vi "MGI VI Scripting Pattern.vi"   [LabVIEW 2016]
doc: "Pattern for scripting VI's to make them more organized and therefore readable.\n\nAuthor: David A. Moore\nsupport@mooregoodideas.com\nwww.mooregoodideas.com\n\nCopyright (c) 2013, Moore Good Ideas, Inc.\n\nAll rights reserved.\n\nRedistribution and use in source and binary forms, with or without modification, are permitted provided that the following conditions are met:\n\n * Redistributions of source code must retain the above copyright notice, this list of conditions and the following disclaimer.\n * Redistributions in binary form must reproduce the above copyright notice, this list of conditions and the following disclaimer in the documentation and/or other materials provided with the distribution.\n * Neither the name of Moore Good Ideas, Inc. nor the names of its contributors may be used to endorse or promote products derived from this software without specific prior written permission.\n\nTHIS SOFTWARE IS PROVIDED BY THE COPYRIGHT HOLDERS AND CONTRIBUTORS \"AS IS\" AND ANY EXPRESS OR IMPLIED WARRANTIES, INCLUDING, BUT NOT LIMITED TO, THE IMPLIED WARRANTIES OF MERCHANTABILITY AND FITNESS FOR A PARTICULAR PURPOSE ARE DISCLAIMED. IN NO EVENT SHALL THE COPYRIGHT OWNER OR CONTRIBUTORS BE LIABLE FOR ANY DIRECT, INDIRECT, INCIDENTAL, SPECIAL, EXEMPLARY, OR CONSEQUENTIAL DAMAGES (INCLUDING, BUT NOT LIMITED TO, PROCUREMENT OF SUBSTITUTE GOODS OR SERVICES; LOSS OF USE, DATA, OR PROFITS; OR BUSINESS INTERRUPTION) HOWEVER CAUSED AND ON ANY THEORY OF LIABILITY, WHETHER IN CONTRACT, STRICT LIABILITY, OR TORT (INCLUDING NEGLIGENCE OR OTHERWISE) ARISING IN ANY WAY OUT OF THE USE OF THIS SOFTWARE, EVEN IF ADVISED OF THE POSSIBILITY OF SUCH DAMAGE."
types:
  T1 = enum16{"<name used in case labels and error messages>"}
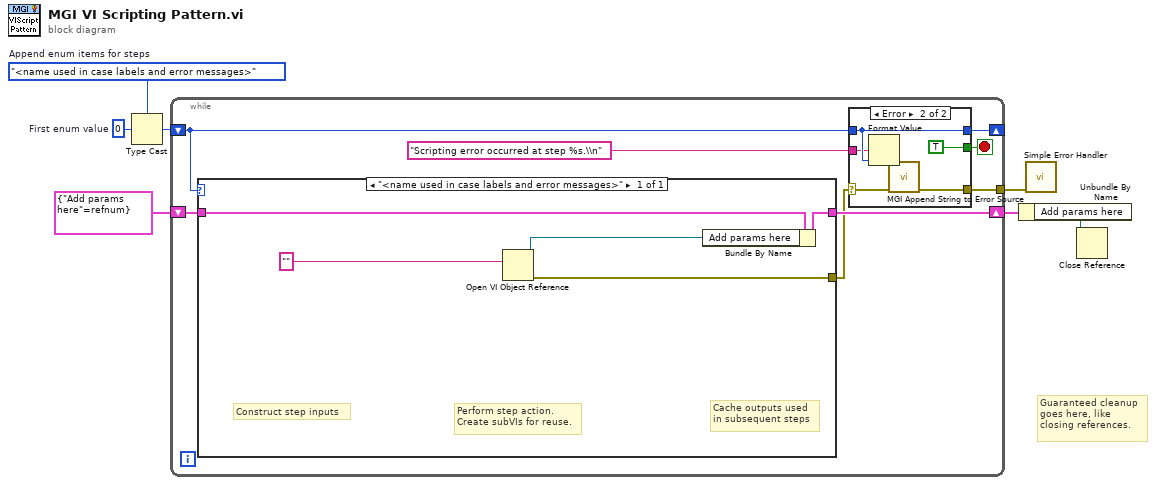
[diagram p0: block diagram]
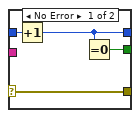
[diagram p2: hidden frame]
diagram:
  w6 = u16 0  # First enum value
  w5 = T1."<name used in case labels and error messages>"  # Append enum items for steps
  # "Guaranteed cleanup\ngoes here, like\nclosing references."
  n1 = Type Cast(type=w5, x=w6) -> (*(type *) &x=w4:T1)
  n2 = while {
    shift-right: [w14] -> w7
    shift-left: cluster{"Add params here":refnum<vi>} {"Add params here"=refnum} ("Arguments") -> [w15]
    shift-right: [w11] -> _
    shift-left: w4 -> [w12]
    tunnel: [w8] -> w1
    stop <- w10 stop-if-true
    n3 = case shown="\"<name used in case labels and error messages>\"" w12 {
      tunnel: w15 -> [w30]
      tunnel: [w29] -> w14
      tunnel: [w28] -> w13
      frame "<name used in case labels and error messages>" {
        # "Cache outputs used\nin subsequent steps"
        # "Perform step action.\nCreate subVIs for reuse."
        # "Construct step inputs"
        n4 = Open VI Object Reference(10:"" ("name/order")) -> (0:w28:errorcluster, 3:w27:refnum<vi>)  [unwired: 3 in]
        n5 = Bundle By Name(cluster=w30, "Add params here"=w27) -> (w29:cluster{"Add params here":refnum<vi>})
      }
    }
    n6 = case shown="Error" w13 {
      selector: w13 -> [w16 w21]
      tunnel: w12 -> [w19 w24]
      tunnel: [w18 w24] -> w11
      tunnel: [w17 TRUE] -> w10
      tunnel: "Scripting error occurred at step %s.\\n" ("format string") -> [_ w23]
      tunnel: [w16 w20] -> w8
      frame No Error {
        n7 = Increment(x=w19) -> (x+1=w18:T1)
        n8 = Equal To 0?(x=w18) -> (x = 0?=w17:bool)
      }
      frame Error {
        n9 = Format Value(format string=w23, value (0)=w24) -> (output string=w22:string)  [unwired: 1 in]
        n10 = call <userlib>:"MGI Append String to Error Source.vi"("Error In"=w21, "String to Append"=w22) -> ("Error Out"=w20:errorcluster)  [unwired: 9 in]
      }
    }
  }
  n11 = Unbundle By Name(w7) -> ("Add params here"=w2:refnum<vi>)
  n12 = call <vilib>:"Simple Error Handler.vi"("error in (no error)"=w1) -> ()  [unwired: 4 in, 5 out]
  n13 = Close Reference(reference=w2) -> ()  [unwired: 1 in, 1 out]
